vi "Generate INSERT SQL Query.vi"(8 "error in (no error)":errorcluster, 10 "Overlappping Records":refnum<class "Statement.lvclass">, 11 "Importing Transactions":refnum<class "Statement.lvclass">) -> (0 "error out":errorcluster, 1 "Num Recs to Insert":i32, 3 "INSERT Query":string)   [LabVIEW 2018, in "Statement.lvclass"]
uses:
  Statement.lvclass
  Statement.lvclass/Statement.ctl
  Transaction/Transaction.lvclass
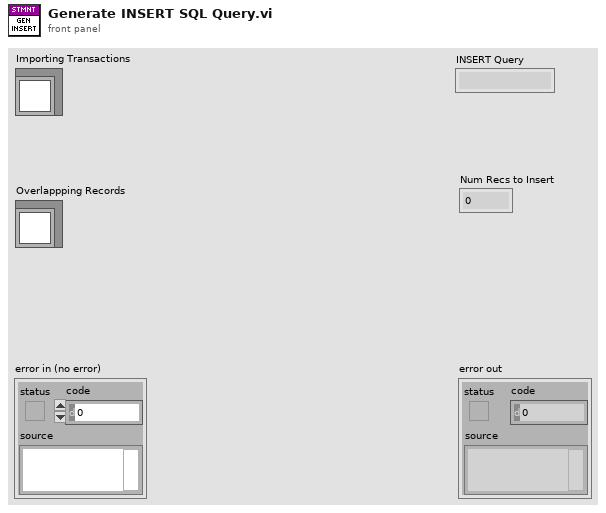
[diagram p1: front panel]
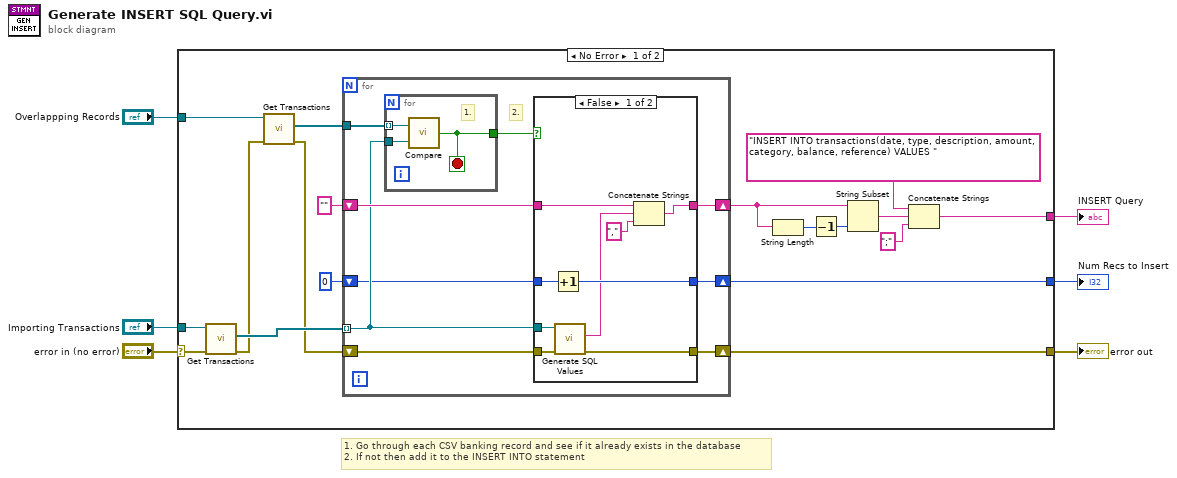
[diagram p0: block diagram]
diagram:
  # "1. Go through each CSV banking record and see if it already exists in the database\n2. If not then add it to the INSERT INTO statement"
  n1 = case shown="No Error" "error in (no error)" {
    selector: "error in (no error)" -> [w13 w49]
    tunnel: [w12 w49] -> w5
    tunnel: "Importing Transactions" -> [w14 _]
    tunnel: [w11 _] -> w3
    tunnel: [w10 _] -> w2
    tunnel: "Overlappping Records" -> [w9 _]
    frame No Error {
      n2 = call "Get Transactions.vi"("error in (no error)"=w13, "Statement in"=w14) -> ("error out"=w8:errorcluster, "Transactions"=w22:refnum<class "Transaction.lvclass">[])  [unwired: 7 in, 1 out]
      n3 = call "Get Transactions.vi"("error in (no error)"=w8, "Statement in"=w9) -> ("error out"=w20:errorcluster, "Transactions"=w21:refnum<class "Transaction.lvclass">[])  [unwired: 7 in, 1 out]
      n4 = for {
        tunnel: w22 -> [w28] mode=indexing
        shift-right: [w32] -> w12
        shift-left: w20 -> [w33]
        shift-right: [w31] -> w15
        shift-left: "" -> [w30]
        tunnel: w21 -> [w29]
        shift-right: [w26] -> w10
        shift-left: 0 -> [w27]
        # "2."
        n5 = for {
          tunnel: w29 -> [w46] mode=indexing
          tunnel: w28 -> [w47]
          tunnel: [w48] -> w25
          stop <- w48 stop-if-true
          # "1."
          n6 = call "Compare.vi"("Transaction y"=w47, "Transaction x"=w46) -> ("Equal?"=w48:bool)
        }
        n7 = case shown="False" w25 {
          tunnel: w33 -> [w37 w44]
          tunnel: [w36 w44] -> w32
          tunnel: [w42 w45] -> w31
          tunnel: w30 -> [w41 w45]
          tunnel: w28 -> [w34 _]
          tunnel: w27 -> [w39 w43]
          tunnel: [w38 w43] -> w26
          frame False {
            n8 = Increment(x=w39) -> (x+1=w38:i32)
            n9 = call-dynamic "Generate SQL Values.vi"("error in (no error)"=w37, "Transaction in"=w34) -> ("error out"=w36:errorcluster, "SQL Values"=w35:string)  [unwired: 7 in, 1 out]
            n10 = Concatenate Strings(w41, w35, "," ("string")) -> (w42:string)
          }
          frame True {
          }
        }
      }
      n11 = String Length(string=w15) -> (length=w17:i32)
      n12 = Decrement(x=w17) -> (x-1=w18:i32)
      n13 = String Subset(string=w15, length (rest)=w18) -> (substring=w19:string)  [unwired: 1 in]
      n14 = Concatenate Strings("INSERT INTO transactions(date, type, description, amount, category, balance, reference) VALUES ", w19, ";" ("string")) -> (w11:string)
    }
    frame Error {
    }
  }
  "error out" <- w5
  "INSERT Query" <- w3
  "Num Recs to Insert" <- w2
